vi "Set Range Controls.vi"(10 "Ranges":T1, 11 "Reference Array":refnum<vi>[](array[refnum])) -> ()   [LabVIEW 2018, in "NI PXI-4110 Programmable Power Supply Custom Device.lvlib"]
uses:
  NI PXI-4110 Programmable Power Supply Custom Device.lvlib
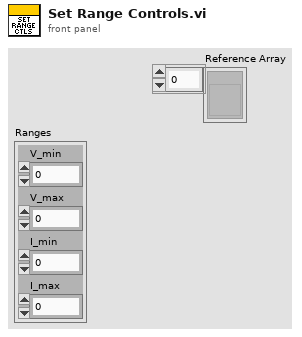
[diagram p1: front panel]
types:
  T1 = cluster{"V_min":dbl, "V_max":dbl, "I_min":dbl, "I_max":dbl}
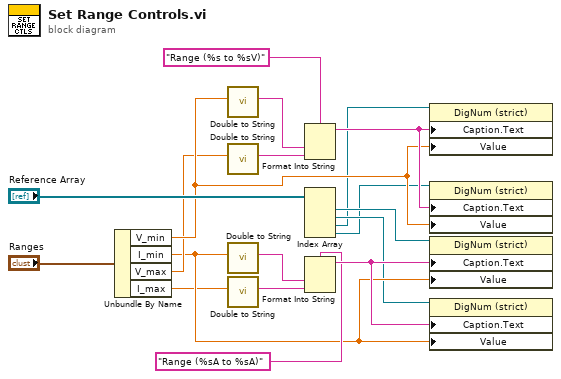
[diagram p0: block diagram]
diagram:
  n1 = Unbundle By Name("Ranges") -> ("V_min"=w12:dbl, "I_min"=w8:dbl, "V_max"=w10:dbl, "I_max"=w7:dbl)
  n2 = call "Double to String.vi"("Double In"=w12) -> ("String Value"=w11:string)  [unwired: 10 in]
  n3 = call "Double to String.vi"("Double In"=w10) -> ("String Value"=w9:string)  [unwired: 10 in]
  n4 = call "Double to String.vi"("Double In"=w8) -> ("String Value"=w6:string)  [unwired: 10 in]
  n5 = call "Double to String.vi"("Double In"=w7) -> ("String Value"=w5:string)  [unwired: 10 in]
  n6 = Format Into String(format string="Range (%s to %sV)" ("Caption.Text"), w11, w9) -> (resulting string=w17:string)  [unwired: 2 in, 1 out]
  n7 = Index Array(array="Reference Array") -> (element #1=w4:refnum<vi>, element #2=w3:refnum<vi>, element #3=w2:refnum<vi>, element #4=w1:refnum<vi>)  [unwired: 4 in]
  n8 = Format Into String(format string="Range (%sA to %sA)" ("Caption.Text"), w6, w5) -> (resulting string=w18:string)  [unwired: 2 in, 1 out]
  n9 = property on="Property Node" class="DigNum (strict)"(reference=w2, "Caption.Text"=w17, "Value"=w12) -> ()  [unwired: 1 in, 2 out]
  n10 = property on="Property Node" class="DigNum (strict)"(reference=w1, "Caption.Text"=w17, "Value"=w12) -> ()  [unwired: 1 in, 2 out]
  n11 = property on="Property Node" class="DigNum (strict)"(reference=w4, "Caption.Text"=w18, "Value"=w8) -> ()  [unwired: 1 in, 2 out]
  n12 = property on="Property Node" class="DigNum (strict)"(reference=w3, "Caption.Text"=w18, "Value"=w8) -> ()  [unwired: 1 in, 2 out]
